vi "QAB Actuators FPGA Old.vi"() -> ()   [LabVIEW 2017]
uses:
  <vilib>/Platform/TimedLoop/XDataNode/timing_clust.ctl
  <vilib>/Platform/TimedLoop/XDataNode/nitl_modes.ctl
  <vilib>/Platform/TimedLoop/XDataNode/wakeup.ctl
  <vilib>/rvi/Emulation/niFpgaGetClockAttributes.vi
  <vilib>/rvi/Emulation/niFpgaSctlEmulationGetInTimedLoop.vi
  <vilib>/rvi/Emulation/niFpgaEmulationReportErrorSimple.vi
  <vilib>/rvi/eio/common/nirviEmuTemplateMethod_errors.vi
  <vilib>/rvi/Emulation/niFpgaCriticalErrorInLSC.vi
  <vilib>/rvi/Emulation/niFpgaEmulationIsFPGAContextNoSignature.vi
  <vilib>/rvi/DataTransferAndStorage/Container/Common/niFpgaContainerGetUniqueNameForEmu.vi
  <vilib>/rvi/Memory/Memory_Emulation/niFpgaMemoryEmulationCacheClearOnFirstRun.vi
  <vilib>/rvi/Memory/Memory_Emulation/nirvimemoryEmulationManagerCache_MakeExclusive.vi
  <vilib>/rvi/Memory/Memory_Emulation/niFpgaMemoryEmulationValidateCache.vi
  <vilib>/rvi/Memory/Memory_Emulation/nirvimemoryEmulationManagerCache_InsertValue.vi
  <vilib>/Utility/error.llb/Clear Errors.vi
  <vilib>/rvi/Memory/Memory_Emulation/nirvimemoryEmulationManagerCache_ReleaseExclusive.vi
  <vilib>/rvi/Memory/Memory_Emulation/nirvimemoryEmulationManagerCache_GetValue.vi
  <vilib>/rvi/Memory/Memory_Emulation/nirvimemoryEmulationManagerCache_SetValue.vi
  <vilib>/rvi/Emulation/niFpgaProcessEmulError.vi
  <vilib>/rvi/DataTransferAndStorage/Container/Common/niFpgaContainerSetEmuInfo.vi
  <vilib>/rvi/eio/common/nirviEmuReportErrorAndStop.vi
  <vilib>/eio/EIONode/EIONode.xnode
  <vilib>/rvi/DataTransferAndStorage/Container/XNode/niFpgaContainer.xnode
  <vilib>/rvi/DataTransferAndStorage/Register/Emulation/niFpgaRegisterEmulation.vi
  <vilib>/Platform/TimedLoop/XDataNode/XDataNode.xnode
  <vilib>/rvi/LocalResourceManager/LocalResourceManager.xnode
  <vilib>/Platform/TimedLoop/XDataNode/XDNodeRunTimeDep.lvlib
panel:
  out "BLDC Motor Tach Ticks":u32
  in  "DC Motor PWM Dir":bool
  in  "BLDC PWM (0-1)":sgl
  in  "Servo Period (1-2ms)":sgl
  out "DC Motor Tach Ticks":u32
  in  "Stepper Control 4":bool
  in  "Stepper Control 3":bool
  in  "Stepper Control 2":bool
  in  "Stepper Control 1":bool
  in  "LED Servo":bool
  in  "LED Stepper":bool
  in  "LED BLDC":bool
  in  "LED DC Motor":bool
  in  "LED Status":bool
  in  "DC Motor Linear Amplifier Enable":bool
  in  "DC Motor PWM (0-1)":sgl
  out "User Button":bool
  out "Power -15V":sgl
  out "Power +15V":sgl
  out "Power +5V":sgl
  out "Power +3.3V":sgl
  out "DC Motor Filtered Current":sgl
  in  "BLDC Drive Phase C":enum16{"H", "L", "Z"}(ring)
  in  "BLDC Drive Phase B":enum16{"H", "L", "Z"}(ring)
  in  "BLDC Drive Phase A":enum16{"H", "L", "Z"}(ring)
  in  "BLDC Encoder Reset":bool
  in  "BLDC Encoder Reset Value":i32
  out "BLDC Encoder Counter":i32
  out "BLDC Encoder RAW A/B/C":fxp<+,3,3> format="%02b"
  in  "LED3:0":fxp<+,4,4> format="%04b"
  in  "DC Linear Amplifier Value (+/-10)":sgl format="%#_17g"
  # "System"
  # "DC Motor"
  # "BLDC"
  # "Stepper"
  # "Servo"
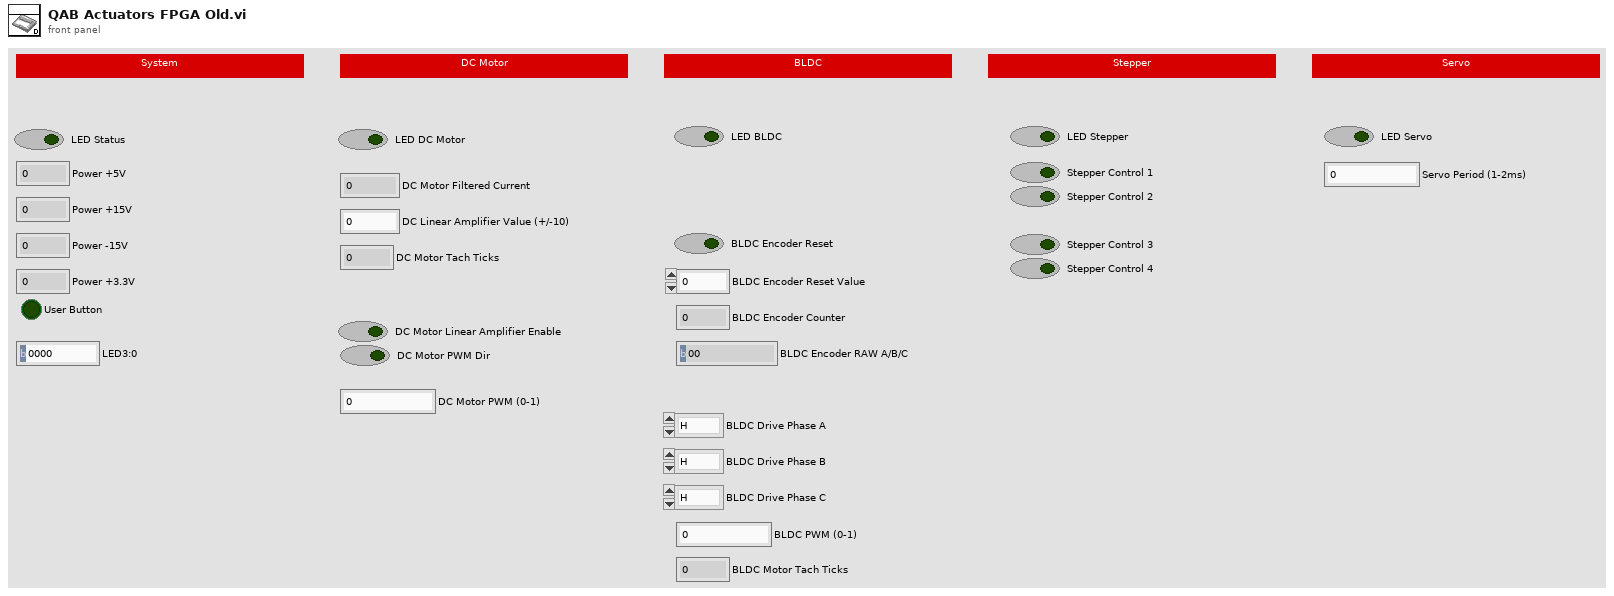
[diagram p1: front panel]
types:
  T1 = typedef "XDNodeRunTimeDep.lvlib/timing_clust.ctl" = cluster{"Expected End [f-1]":u64, "Actual End [f-1]":u64, "Finished Late? [f-1]":bool, "Expected End [i-1]":u64, "Actual End [i-1]":u64, "Finished Late? [i-1]":bool, "Expected Start [i]":u64, "Actual Start [i]":u64, "Expected Start [f]":u64, "Actual Start [f]":u64, "Source Name":string, "Structure Name":string, "Period":i64, "Deadline":i64, "Offset":i64, "Start":i64, "Priority":i32, "Timeout":i32, "Mode":T2, "Wakeup Reason":T3, "Error":errorcluster, "Source Type":string, "Secondary Source Type":string, "Global End Time":u64, "Global Start Time":u64, "Frame Duration":u64, "Iteration Duration":u64, "Assigned CPU":i32, "I/O Scan Engine Mode":u32}
  T2 = typedef "XDNodeRunTimeDep.lvlib/nitl_modes.ctl" = enum32{"No Change", "Process missed periods, maintain original phase", "Discard missed periods, maintain original phase", "Process missed periods, ignore original phase", "Discard missed periods, ignore original phase"}
  T3 = typedef "XDNodeRunTimeDep.lvlib/wakeup.ctl" = enum32{"Normal", "Aborted", "Asynchronous wakeup", "Timing source error", "Timed loop error", "Timeout"}
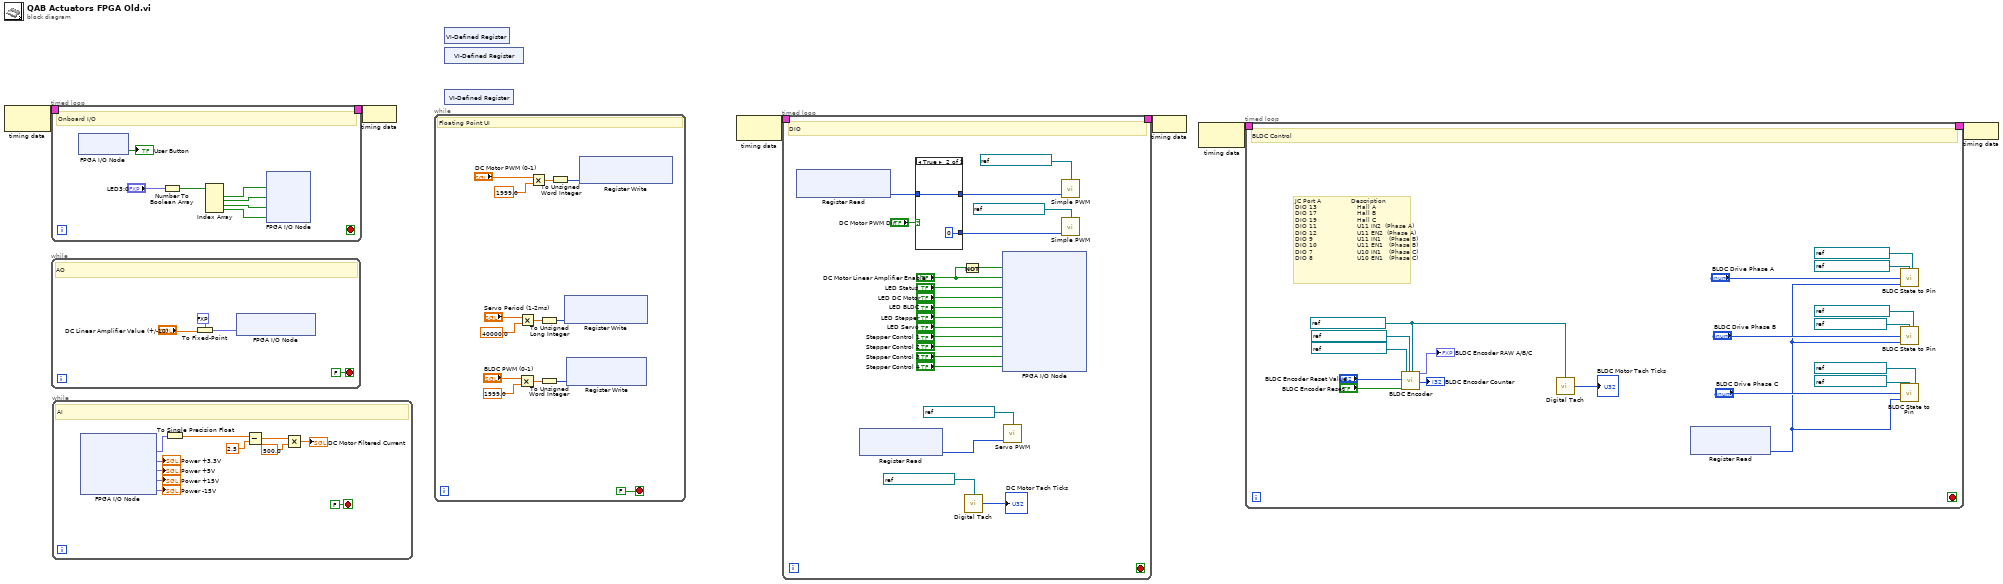
[diagram p0: block diagram]
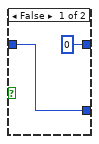
[diagram p2: hidden frame]
diagram:
  n1 = node-c288() -> (w6:T1)  [unwired: 1 in]
  n2 = timed-loop {
    timing: w6 -> [_]
    timing-out: [_] -> w5
    stop <- _ stop-if-true
    # "Onboard I/O"
    n3 = xnode "FPGA I/O Node"() -> ("Button0"=→"User Button":bool)  [unwired: 1 in, 1 out]
    n4 = Number To Boolean Array(number="LED3:0") -> (Boolean array=w12:bool[])
    n5 = Index Array(array=w12) -> (element #1=w11:bool, element #2=w10:bool, element #3=w9:bool, element #4=w8:bool)  [unwired: 4 in]
    n6 = xnode "FPGA I/O Node"("LED0"=w11, "LED1"=w10, "LED2"=w9, "LED3"=w8) -> ()  [unwired: 4 in, 4 out]
  }
  n7 = while {
    stop <- FALSE stop-if-true
    # "AO"
    n8 = To Fixed-Point(fixed-point type=fxp<+/-,20,5> 0.0 ("ConnectorA/AO0"), number="DC Linear Amplifier Value (+/-10)") -> (fixed-point=w16:fxp<+/-,20,5>)
    n9 = xnode "FPGA I/O Node"("ConnectorA/AO0"=w16) -> ()  [unwired: 1 in, 1 out]
  }
  n10 = while {
    stop <- FALSE stop-if-true
    # "AI"
    n11 = xnode "FPGA I/O Node"() -> ("ConnectorA/AI0"=w25:fxp<+/-,24,5>, "ConnectorB/AI4"=→"Power +3.3V":fxp<+/-,24,5>, "ConnectorB/AI5"=→"Power +5V":fxp<+/-,24,5>, "ConnectorB/AI6"=→"Power +15V":fxp<+/-,24,5>, "ConnectorB/AI7"=→"Power -15V":fxp<+/-,24,5>)  [unwired: 5 in, 5 out]
    n12 = To Single Precision Float(number=w25) -> (single precision float=w20:sgl)
    n13 = Subtract(x=w20, y=sgl 2.5) -> (x-y=w23:sgl)
    n14 = Multiply(x=w23, y=sgl 500.0) -> (x*y=→"DC Motor Filtered Current":sgl)
  }
  n15 = node-c288(w5) -> ()
  n16 = while {
    stop <- FALSE stop-if-true
    # "Floating Point UI"
    n17 = Multiply(x="BLDC PWM (0-1)", y=sgl 1999.0) -> (x*y=w34:sgl)
    n18 = Multiply(x="Servo Period (1-2ms)", y=sgl 40000.0) -> (x*y=w41:sgl)
    n19 = Multiply(x="DC Motor PWM (0-1)", y=sgl 1999.0) -> (x*y=w39:sgl)
    n20 = To Unsigned Word Integer(number=w34) -> (unsigned 16bit integer=w31:u16)
    n21 = To Unsigned Long Integer(number=w41) -> (unsigned 32bit integer=w35:u32)
    n22 = To Unsigned Word Integer(number=w39) -> (unsigned 16bit integer=w36:u16)
    n23 = xnode ("Register Write")("Data"=w35) -> ()  [unwired: 1 in, 1 out]
    n24 = xnode ("Register Write")("Data"=w31) -> ()  [unwired: 1 in, 1 out]
    n25 = xnode ("Register Write")("Data"=w36) -> ()  [unwired: 1 in, 1 out]
  }
  n26 = xnode "VI-Defined Register"() -> ()  [unwired: 1 out]
  n27 = xnode "VI-Defined Register"() -> ()  [unwired: 1 out]
  n28 = xnode "VI-Defined Register"() -> ()  [unwired: 1 out]
  n29 = node-c288() -> (w2:T1)  [unwired: 1 in]
  n30 = timed-loop {
    timing: w2 -> [_]
    timing-out: [_] -> w1
    stop <- _ stop-if-true
    # "DIO"
    n31 = xnode ("Register Read")() -> ("Data"=w46:u16)  [unwired: 1 in, 1 out]
    n32 = xnode ("Register Read")() -> ("Data"=w48:u32)  [unwired: 1 in, 1 out]
    n33 = case shown="True" "DC Motor PWM Dir" {
      tunnel: w46 -> [w66 w68]
      tunnel: [u16 0 ("Data") w68] -> w45
      tunnel: [w66 u16 0 ("Data")] -> w44
      frame False {
      }
      frame True {
      }
    }
    n34 = Not(x="DC Motor Linear Amplifier Enable") -> (.not. x?=w50:bool)
    n35 = call "Digital Tach.vi"("Input Pin"=refnum<k21> "ConnectorA/DIO5" ("Drive Pin")) -> ("Tach Ticks"=→"DC Motor Tach Ticks":u32)  [unwired: 3 in]
    n36 = xnode "FPGA I/O Node"("ConnectorA/DIO2"=w50, "ConnectorA/DIO6"="DC Motor Linear Amplifier Enable", "ConnectorA/DIO16"="LED Status", "ConnectorA/DIO18"="LED DC Motor", "ConnectorB/DIO18"="LED BLDC", "ConnectorB/DIO16"="LED Stepper", "ConnectorB/DIO19"="LED Servo", "ConnectorB/DIO5"="Stepper Control 1", "ConnectorB/DIO7"="Stepper Control 2", "ConnectorB/DIO9"="Stepper Control 3", "ConnectorB/DIO11"="Stepper Control 4") -> ()  [unwired: 11 in, 11 out]
    n37 = call "Servo PWM.vi"("Drive Pin"=refnum<k21> "ConnectorB/DIO3", "Duty Cycle"=w48) -> ()  [unwired: 3 in]
    n38 = call "Simple PWM.vi"("Drive Pin"=refnum<k21> "ConnectorA/DIO0", "Duty Cycle (0-1999)"=w45) -> ()  [unwired: 3 in]
    n39 = call "Simple PWM.vi"("Drive Pin"=refnum<k21> "ConnectorA/DIO3", "Duty Cycle (0-1999)"=w44) -> ()  [unwired: 3 in]
  }
  n40 = node-c288(w1) -> ()
  n41 = node-c288() -> (w4:T1)  [unwired: 1 in]
  n42 = timed-loop {
    timing: w4 -> [_]
    timing-out: [_] -> w3
    stop <- _ stop-if-true
    w71 = refnum<k21> "ConnectorA/DIO19" ("C")
    # "JC Port A               Description\nDIO 13\t\t                  Hall A\nDIO 17\t\t                  Hall B\nDIO 19\t\t                  Hall C\nDIO 11\t\t                  U11 IN2  (Phase A)\nDIO 12\t\t                  U11 EN2  (Phase A)\nDIO 9\t\t                   \tU11 IN1    (Phase B)\nDIO 10\t\t                  U11 EN1   (Phase B)\nDIO 7\t\t                    U10 IN1    (Phase C)\nDIO 8\t\t                    U10 EN1   (Phase C)"
    # "BLDC Control"
    n43 = call "BLDC Encoder.vi"("Encoder Reset Value"="BLDC Encoder Reset Value", "Encoder Reset"="BLDC Encoder Reset", "A"=refnum<k21> "ConnectorA/DIO13" ("B"), "B"=refnum<k21> "ConnectorA/DIO17" ("A"), "C"=w71) -> ("Encoder RAW A/B/C"=→"BLDC Encoder RAW A/B/C":fxp<+,3,3>, "Encoder Counter"=→"BLDC Encoder Counter":i32)  [unwired: 12 in, 1 out]
    n44 = call "Digital Tach.vi"("Input Pin"=w71) -> ("Tach Ticks"=→"BLDC Motor Tach Ticks":u32)  [unwired: 3 in]
    n45 = xnode ("Register Read")() -> ("Data"=w73:u16)  [unwired: 1 in, 1 out]
    n46 = call "BLDC State to Pin.vi"("Enable"=refnum<k21> "ConnectorA/DIO12", "Drive Pin"=refnum<k21> "ConnectorA/DIO11", "Compare Value"=w73, "State"="BLDC Drive Phase A") -> ()  [unwired: 1 in]
    n47 = call "BLDC State to Pin.vi"("Enable"=refnum<k21> "ConnectorA/DIO10", "Drive Pin"=refnum<k21> "ConnectorA/DIO9", "Compare Value"=w73, "State"="BLDC Drive Phase B") -> ()  [unwired: 1 in]
    n48 = call "BLDC State to Pin.vi"("Enable"=refnum<k21> "ConnectorA/DIO8", "Drive Pin"=refnum<k21> "ConnectorA/DIO7", "Compare Value"=w73, "State"="BLDC Drive Phase C") -> ()  [unwired: 1 in]
  }
  n49 = node-c288(w3) -> ()
